vi "Sub_OBS.vi"(6 "Yin":dbl, 9 "DutyCycle_OBS":dbl, 10 "k_OBS":dbl, 11 "b_OBS":dbl=1.0) -> (1 "x2hat":dbl, 2 "x1hat":dbl)   [LabVIEW 2019]
uses:
  <vilib>/Simulation/Implementation/Shared/SIMSCR Execution Mode.ctl
  <vilib>/Simulation/Scripting/Companion Diagram/SimConfigNode/SimParams.ctl
  <vilib>/Simulation/Scripting/Companion Diagram/SimConfigNode/_simSolvers.ctl
  <vilib>/Simulation/Param Hierarchy/Typedefs/SIMPH Param Control Actions.ctl
  <vilib>/Simulation/Implementation/Shared/SIM limit type.ctl
  <vilib>/Simulation/Implementation/Shared/NILVSim_ParamChanged.vi
  <vilib>/Simulation/Implementation/Shared/NILVSIM_BeginStep.vi
  <vilib>/Simulation/SignalArithmetic/Implementation/NILVSim Gain.llb/SIM Gain (scalar).vi
  <vilib>/Simulation/ContinuousLinear/Implementation/NILVSim Integrator new.llb/SIM Integrator distributor (scalar).vi
  <vilib>/Simulation/ContinuousLinear/Implementation/NILVSim Integrator new.llb/SIM Integrator collector (scalar).vi
  <vilib>/Simulation/Implementation/Shared/NILVSim_Manager.vi
  <vilib>/Utility/error.llb/Clear Errors.vi
  <vilib>/Simulation/Implementation/Shared/NILVSim_FinalizeModel.vi
  <vilib>/Simulation/Implementation/Shared/SIM Unbundle Sim Info.vi
  <vilib>/Simulation/Implementation/Shared/SIMSH Read Queue.vi
  <vilib>/Simulation/Implementation/Shared/NILVSim_Initialize.vi
  <vilib>/Simulation/Utility/Implementation/NILVSim Get Time and IsAcceptedStep.vi
  <vilib>/Simulation/Implementation/Shared/NILVSim_GetModelError.vi
  <vilib>/Simulation/Implementation/Shared/SIM SimErrorHandler.vi
  <vilib>/Simulation/Implementation/Shared/SIM Bundle Sim Info.vi
  <vilib>/Simulation/Scripting/Companion Diagram/SimConfigNode/SimDog.xnode
  <vilib>/Simulation/Implementation/XNodeFramework/SimXNode/SimX.xnode
  <vilib>/Simulation/ContinuousLinear/Implementation/NILVSim Integrator new.llb/SIM Integrator (scalar).vi
  <vilib>/Simulation/Implementation/Shared/NI_SIM_Implementation.lvlib
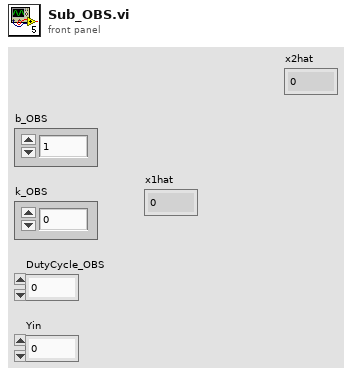
[diagram p1: front panel]
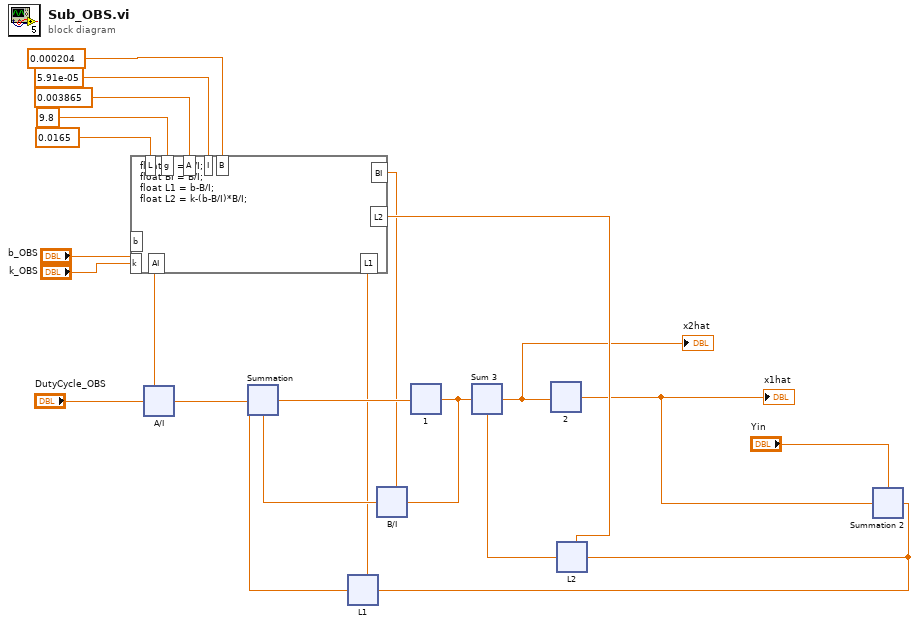
[diagram p0: block diagram]
diagram:
  n1 = formula code="float AI = A/I;\nfloat BI = B/I;\nfloat L1 = b-B/I;\nfloat L2 = k-(b-B/I)*B/I;"("L"=0.0165 ("input variable"), "g"=9.8 ("input variable 2"), "A"=0.003865 ("input variable 3"), "I"=5.91e-05 ("input variable 4"), "B"=0.000204 ("input variable 5"), "b"="b_OBS", "k"="k_OBS") -> ("AI"=w6:dbl, "BI"=w11:dbl, "L1"=w3:dbl, "L2"=w22:dbl)
  n2 = xnode "A/I"("gain"=w6, "input"="DutyCycle_OBS") -> ("output"=w17:dbl)  [unwired: 2 in]
  n3 = xnode "Summation"("Operand1"=w17, "Operand2"=w2, "Operand3"=w8) -> ("Result"=w18:dbl)
  n4 = xnode "1"("input"=w18) -> ("output"=w21:dbl)  [unwired: 9 in, 2 out]
  n5 = xnode "B/I"("gain"=w11, "input"=w21) -> ("output"=w8:dbl)  [unwired: 2 in]
  n6 = xnode "L1"("gain"=w3, "input"=w19) -> ("output"=w2:dbl)  [unwired: 2 in]
  n7 = xnode "Sum 3"("Operand1"=w21, "Operand2"=w20) -> ("Result"=w1:dbl)
  "x2hat" <- w1
  n8 = xnode "2"("input"=w1) -> ("output"=w10:dbl)  [unwired: 9 in, 2 out]
  "x1hat" <- w10
  n9 = xnode "Summation 2"("Operand1"="Yin", "Operand2"=w10) -> ("Result"=w19:dbl)
  n10 = xnode "L2"("gain"=w22, "input"=w19) -> ("output"=w20:dbl)  [unwired: 2 in]
